vi "Transmit.vi"(8 "error in (no error)":errorcluster, 10 "Transfer Group in":refnum<class "Transfer Group.lvclass">, 11 "UDP Transceiver in":refnum<class "UDP Transceiver.lvclass">) -> (0 "error out":errorcluster, 2 "Transfer Group out":refnum<class "Transfer Group.lvclass">, 3 "UDP Transceiver out":refnum<class "UDP Transceiver.lvclass">)   [LabVIEW 2017, in "UDP.lvlib" / "UDP Transceiver.lvclass"]
uses:
  UDP Transceiver.lvclass
  Builds/Data Sharing Framework/Current/Data Sharing Framework Core/DSF Core.lvlibp/Engine/Classes/Transfer Group/Transfer Group.lvclass
  UDP Transceiver.lvclass/UDP Transceiver.ctl
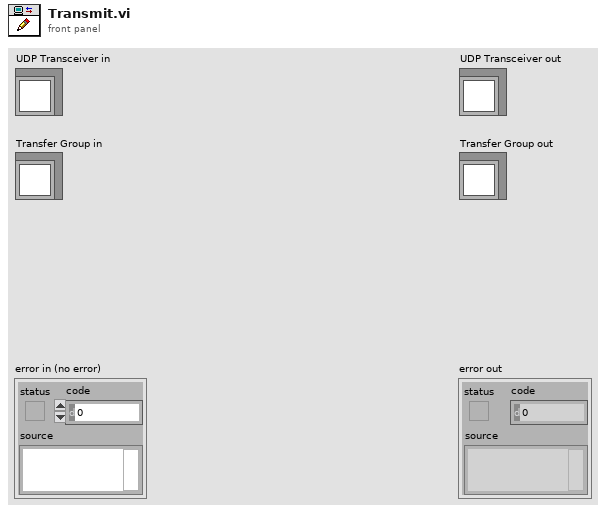
[diagram p1: front panel]
types:
  T1 = typedef "UDP.lvlib/UDP Transceiver.lvclass/Transfer Group Parameters.ctl" = cluster{"Rx":T2, "Tx":T4}
  T2 = typedef "UDP.lvlib/UDP Transceiver.lvclass/Transfer Group Rx Parameters.ctl" = cluster{"Transfers Rx":T3[], "max size":i32}
  T3 = typedef "UDP.lvlib/UDP Transceiver.lvclass/Transfer Rx Parameters.ctl" = cluster{"timeout":i32, "source address":u32, "source port":u16}
  T4 = typedef "UDP.lvlib/UDP Transceiver.lvclass/Transfer Group Tx Parameters.ctl" = cluster{"Transfers Tx":T5[]}
  T5 = typedef "UDP.lvlib/UDP Transceiver.lvclass/Transfer Tx Parameters.ctl" = cluster{"destination port":u16, "destination address":u32}
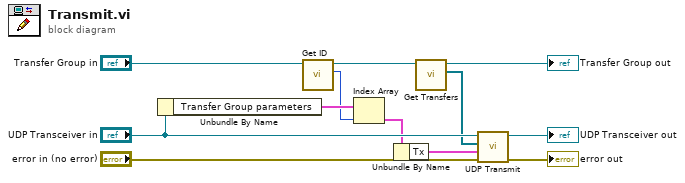
[diagram p0: block diagram]
diagram:
  n1 = Unbundle By Name("UDP Transceiver in") -> ("Transfer Group parameters"=w10:T1[])
  n2 = call "Get ID.vi"("Transfer Group in"="Transfer Group in") -> ("id"=w9:i32, "Transfer Group out"=w11:refnum<class "Transfer Group.lvclass">)  [unwired: 9 in]
  n3 = Index Array(array=w10, index=w9) -> (element=w1:T1)
  n4 = Unbundle By Name(w1) -> ("Tx"=w12:T4)
  n5 = call "Get Transfers.vi"("Transfer Group in"=w11) -> ("Transfers"=w2:refnum<class "Transfer.lvclass">[], "Transfer Group out"=→"Transfer Group out":refnum<class "Transfer Group.lvclass">)  [unwired: 9 in]
  n6 = call "UDP Transmit.vi"("error in (no error)"="error in (no error)", "Tx"=w12, "Transfers"=w2, "UDP Transceiver in"="UDP Transceiver in") -> ("error out"=→"error out":errorcluster, "UDP Transceiver out"=→"UDP Transceiver out":refnum<class "UDP Transceiver.lvclass">)  [unwired: 6 in]
